vi "AutoLand_Approach.vi"(1 "Autoland?":bool, 2 "Step-Approach?":bool) -> (0 "Finished?":bool)   [LabVIEW 2015]
uses:
  D:/LabVIEW for ezAFM/LV-PGC 2019-05a/Special Equipment/ezAFM/NMI Integration Code/ezCommander.dll
  LabVIEW for ezAFM/LV-PGC 2019-05a/Special Equipment/ezAFM/NMI Integration Code/ezCommander.dll
  LabVIEW for ezAFM/LV-PGC 2019-05a/Universal vi's/Global Variables/Globals-EasyAFM.vi
  Globals.vi
panel:
  out "XYZ Motor Position":dbl[](array[numeric])
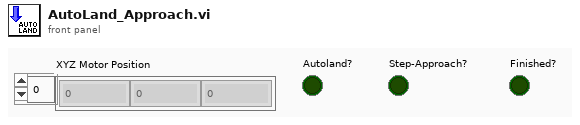
[diagram p1: front panel]
types:
  T1 = enum16{"Read XYZ Motor Position", "Read XYZ Piezo Position", "Read Setpoint", "Begin AutoLand", "Begin AutoLand, Wait till done", "XYZ Motions", "Init Scan (from global settings)", "Start Scan", "Stop Scan"}
  T2 = cluster{"Approach":bool, "Retract":bool, "Up":bool, "Up-Right":bool, "Right":bool, "Up Left":bool}
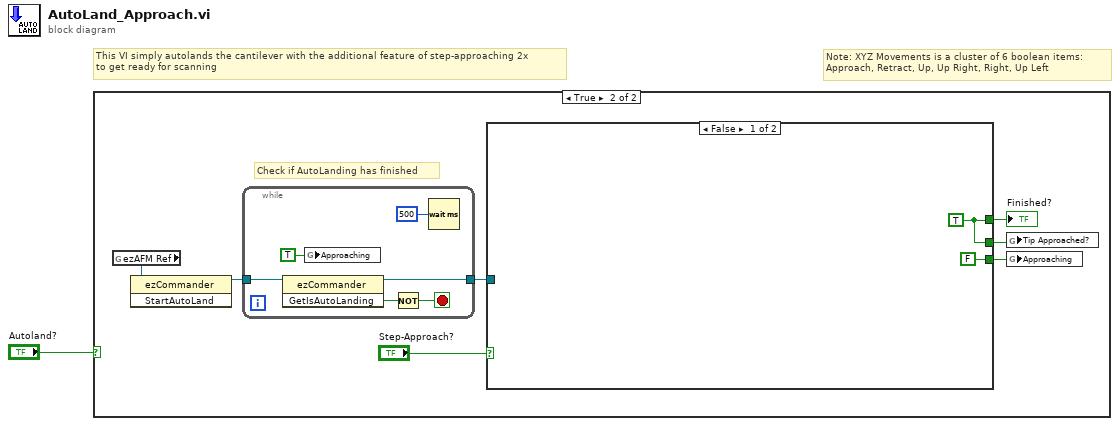
[diagram p0: block diagram]
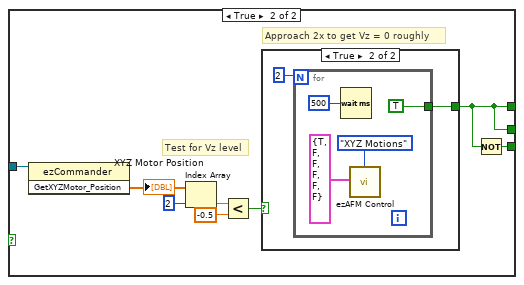
[diagram p3: hidden frame]
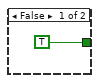
[diagram p4: hidden frame]
diagram:
  # "This VI simply autolands the cantilever with the additional feature of step-approaching 2x\nto get ready for scanning"
  # "Note: XYZ Movements is a cluster of 6 boolean items: \nApproach, Retract, Up, Up Right, Right, Up Left"
  n1 = case shown="True" "Autoland?" {
    frame False {
    }
    frame True {
      # "Check if AutoLanding has finished"
      n2 = global read "Globals-EasyAFM.vi" "ezAFM Ref"() -> (w7:refnum<k24>)
      n3 = invoke class="ezCommander" method="StartAutoLand"(reference=w7) -> (reference out=w8:refnum<k24>)  [unwired: 2 in, 2 out]
      n4 = while {
        tunnel: w8 -> [w31]
        tunnel: [w27] -> w6
        stop <- w30 stop-if-true
        n5 = invoke class="ezCommander" method="GetIsAutoLanding"(reference=w31) -> (reference out=w27:refnum<k24>, "GetIsAutoLanding"=w29:bool)  [unwired: 2 in, 1 out]
        n6 = global write "Globals.vi" "Approaching"(TRUE ("Approaching")) -> ()
        n7 = Not(x=w29) -> (.not. x?=w30:bool)
        n8 = Wait (ms)(milliseconds to wait=u32 500) -> ()  [unwired: 1 out]
      }
      n9 = case shown="False" "Step-Approach?" {
        tunnel: w6 -> [_ w15]
        tunnel: [w9 w11] -> w4
        tunnel: [FALSE w12] -> w3
        tunnel: [w9 w11] -> w2
        frame False {
          w9 = TRUE
        }
        frame True {
          # "Approach 2x to get Vz = 0 roughly"
          # "Test for Vz level"
          n10 = invoke class="ezCommander" method="GetXYZMotor_Position"(reference=w15) -> ("GetXYZMotor_Position"=w14:dbl[])  [unwired: 2 in, 2 out]
          "XYZ Motor Position" <- w14
          n11 = Index Array(array=w14, index=2) -> (element=w17:dbl)
          n12 = Less?(x=w17, y=-0.5) -> (x < y?=w13:bool)
          n13 = case shown="True" w13 {
            tunnel: [TRUE ("Finished") w20] -> w11
            frame False {
            }
            frame True {
              n14 = for {
                N: 2 -> [_]
                tunnel: [TRUE ("Finished")] -> w20
                n15 = Wait (ms)(milliseconds to wait=u32 500) -> ()  [unwired: 1 out]
                n16 = call "ezAFM Control.vi"("XYZ Movements"=T2 {"Approach"=TRUE, "Retract"=FALSE, "Up"=FALSE, "Up-Right"=FALSE, "Right"=FALSE, "Up Left"=FALSE}, "Mode"=T1."XYZ Motions") -> ()  [unwired: 3 in, 4 out]
              }
            }
          }
          n17 = Not(x=w11) -> (.not. x?=w12:bool)
        }
      }
      "Finished?" <- w4
      n18 = global write "Globals.vi" "Tip Approached?"(w2) -> ()
      n19 = global write "Globals.vi" "Approaching"(w3) -> ()
    }
  }
